vi "SwitchingCameraSendImagesToPCLoop.vi"(8 "error in (no error)":errorcluster, 9 "port":u16=1181, 10 "AutoSwitchCameraName":string="Sequenced Camera") -> ()   [LabVIEW 2019, in "ArgosLib.lvlib"]
doc: "This VI is used to serve images from one or more named cameras on your robot to the dashboard, SmartDashboard, or compatible web browser. Camera name and type info is published using network tables. Connections are on port 1181 by default and the URL for streaming can be found by looking at the network \"camera\"/streams variable. Cameras that are opened and stored in the name registry are automatically published by that name.\n\nThis VI runs in parallel with other code and should be placed in Robot Main or in Periodic Tasks.\n\nThis software is licensed. Open the labview\\readme\\WPI Robotics Library Open Source License.txt file for more information."
uses:
  ArgosLib.lvlib
  <vilib>/Rock Robotics/WPI/Utilities/Refnum Registry Operation.ctl
  <vilib>/Rock Robotics/Network Tables/NT Write String Array.vi
  <vilib>/Rock Robotics/Network Tables/NT Write String.vi
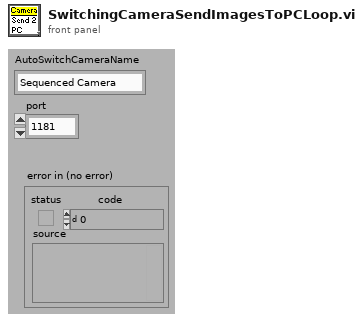
[diagram p1: front panel]
types:
  T1 = enum16{"Standard", "Buffered", "CRLF", "Immediate"}
  T2 = typedef "Refnum Registry Operation.ctl" = enum16{"set", "get", "delete", "get all names", "read name"}
  T3 = cluster{"token string":string, "token string 2":string}[]
  T4 = typedef "WPI_CameraDevRef.ctl" = cluster{"Camera Address":string, "CameraStatus":errorcluster}
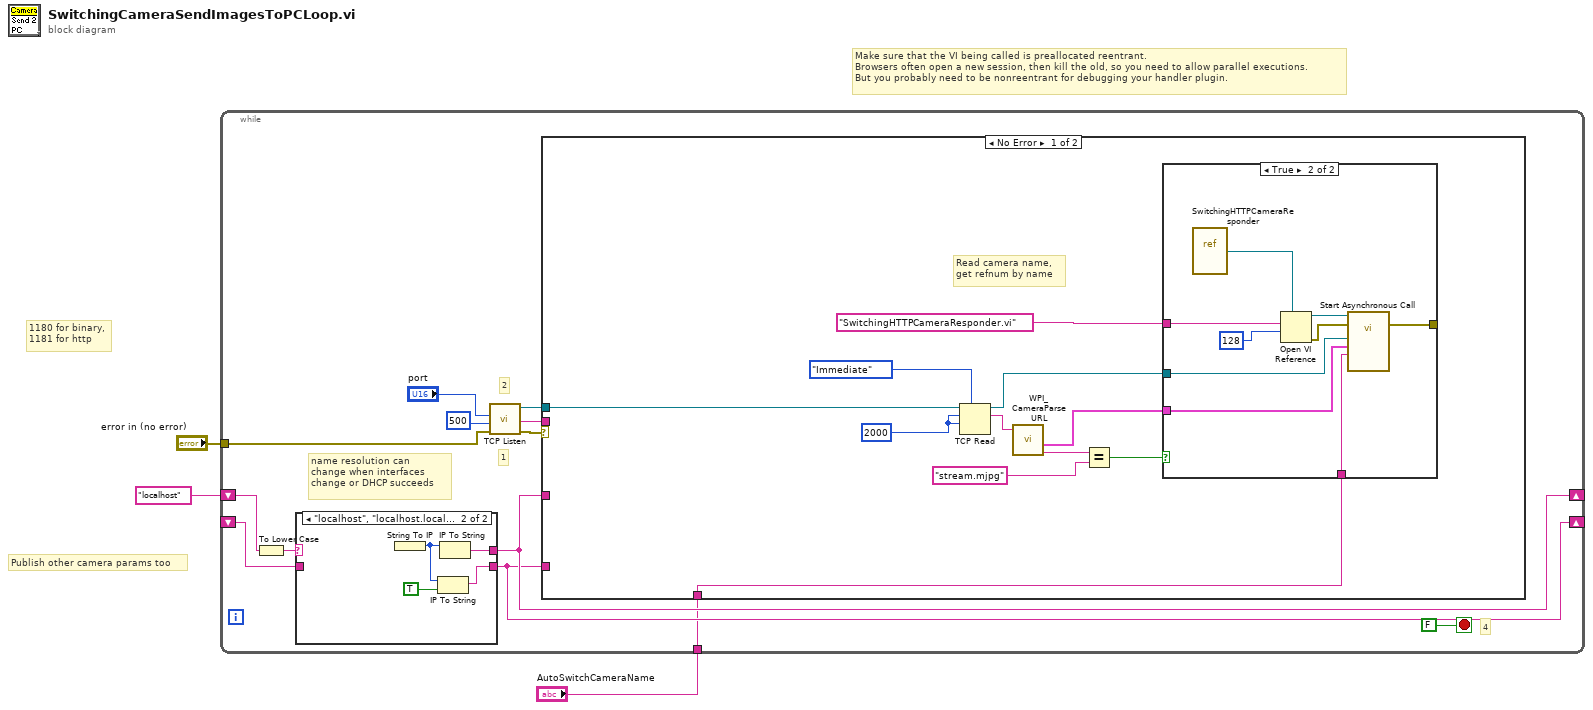
[diagram p0: block diagram]
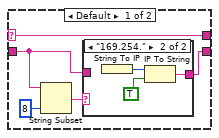
[diagram p2: hidden frame]
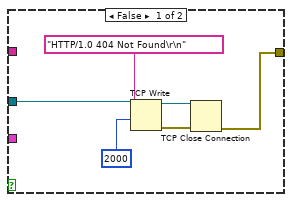
[diagram p4: hidden frame]
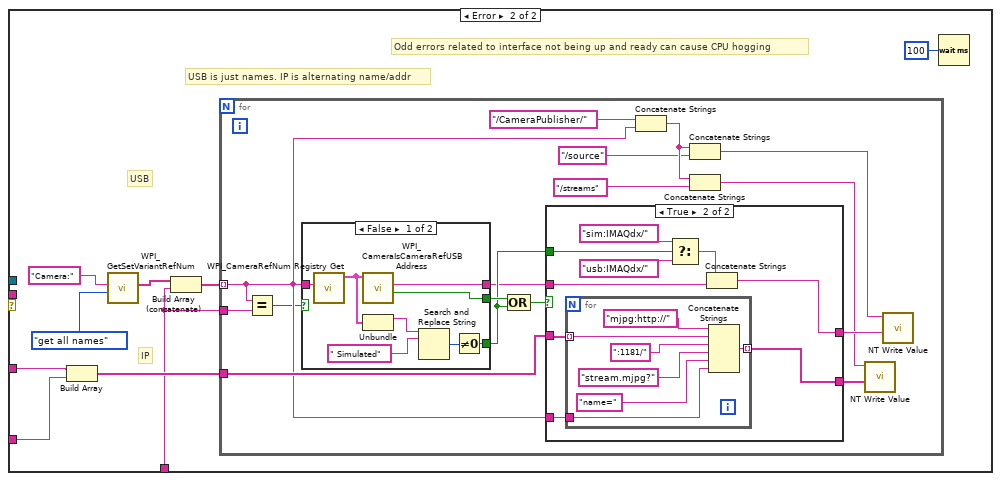
[diagram p5: hidden frame]
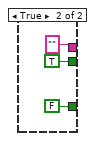
[diagram p6: hidden frame]
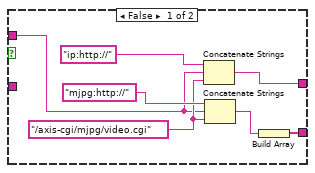
[diagram p7: hidden frame]
diagram:
  # "Make sure that the VI being called is preallocated reentrant.\nBrowsers often open a new session, then kill the old, so you need to allow parallel executions.\nBut you probably need to be nonreentrant for debugging your handler plugin."
  # "Publish other camera params too"
  # "1180 for binary,\n1181 for http"
  n1 = while {
    tunnel: "error in (no error)" -> [w15]
    shift-right: [w7] -> _
    shift-left: "localhost" -> [w8]
    shift-right: [w5] -> _
    shift-left: _ -> [w6]
    tunnel: "AutoSwitchCameraName" -> [w4]
    stop <- FALSE ("status") stop-if-true
    # "name resolution can\nchange when interfaces\nchange or DHCP succeeds"
    # "4"
    # "1"
    # "2"
    n2 = To Lower Case(string=w8) -> (all lower case string=w9:string)
    n3 = case shown="\"localhost\", \"localhost.localdomain\"" w9 {
      selector: w9 -> [w21 _]
      tunnel: [w21 w29] -> w7
      tunnel: w6 -> [w18 _]
      tunnel: [w17 w26] -> w5
      frame Default {
        n4 = String Subset(string=w18, length (rest)=8 ("length (rest)")) -> (substring=w19:string)  [unwired: 1 in]
        n5 = case shown="\"169.254.\"" w19 {
          tunnel: w18 -> [w22 _]
          tunnel: [w22 w23] -> w17
          frame Default {
          }
          frame "169.254." {
            n6 = String To IP() -> (0:w25:u32)  [unwired: 1 in]
            n7 = IP To String(1:TRUE ("dot notation? (F)"), 2:w25) -> (0:w23:string)
          }
        }
      }
      frame "localhost", "localhost.localdomain" {
        n8 = String To IP() -> (0:w27:u32)  [unwired: 1 in]
        n9 = IP To String(1:TRUE ("dot notation? (F)"), 2:w27) -> (0:w26:string)
        n10 = IP To String(2:w27) -> (0:w29:string)  [unwired: 1 in]
      }
    }
    n11 = call <vilib>:"TCP Listen.vi"("error in (no error)"=w15, "timeout ms (wait forever: -1)"=u16 500 ("port"), "port"="port") -> ("error out"=w12:errorcluster, "remote address"=w16:string, "connection ID"=w14:refnum<k5>)  [unwired: 1 in, 5 out]
    n12 = case shown="No Error" w12 {
      tunnel: w16 -> [_ _]
      tunnel: w14 -> [w37 _]
      tunnel: w7 -> [_ w61]
      tunnel: w5 -> [_ w59]
      tunnel: w4 -> [w30 w56]
      frame No Error {
        w38 = 2000
        # "Read camera name,\nget refnum by name"
        n13 = TCP Read(connection ID=w37, bytes to read=w38, 7:T1."Immediate" ("mode (standard)"), 9:w38) -> (connection ID out=w36:refnum<k5>, data out=w31:string)  [unwired: 1 in, 1 out]
        n14 = call <vilib>:"WPI_CameraParse URL.vi"("URL"=w31) -> ("cgi string"=w33:string, "parameters"=w32:T3)  [unwired: 7 in, 2 out]
        n15 = Equal?(x=w33, y="stream.mjpg") -> (x = y?=w35:bool)
        n16 = case shown="True" w35 {
          tunnel: "SwitchingHTTPCameraResponder.vi" -> [_ w55]
          tunnel: w36 -> [w46 w51]
          tunnel: [w41 w49] -> _
          tunnel: w32 -> [_ w48]
          tunnel: w30 -> [_ w47]
          frame False {
            n17 = TCP Write(connection ID=w46, data in="HTTP/1.0 404 Not Found\r\n" ("regular expression"), 9:2000) -> (connection ID out=w45:refnum<k5>, error out=w42:errorcluster)  [unwired: 1 in, 1 out]
            n18 = TCP Close Connection(connection ID=w45, error in (no error)=w42) -> (error out=w41:errorcluster)  [unwired: 2 out]
          }
          frame True {
            n19 = vi-ref "SwitchingHTTPCameraResponder.vi"() -> (w53:refnum<vi>)
            n20 = Open VI Reference(type specifier VI Refnum (for type only)=w53, vi path=w55, options=128) -> (vi reference=w52:refnum<vi>, error out=w50:errorcluster)  [unwired: 3 in]
            n21 = call-by-ref "Start Asynchronous Call"(reference=w52, error in=w50, "Switched Camera Name"=w47, "parameters"=w48, "connection ID"=w51) -> (error out=w49:errorcluster)  [unwired: 9 in, 1 out]
          }
        }
      }
      frame Error {
        # "USB is just names. IP is alternating name/addr"
        # "IP"
        # "USB"
        # "Odd errors related to interface not being up and ready can cause CPU hogging"
        n22 = Build Array(w61, w59) -> (w60:string[])
        n23 = call <vilib>:"WPI_GetSetVariantRefNum.vi"("Operation"=Refnum_Registry_Operation."get all names" ("menu"), "refnum name"="Camera:") -> ("names"=w58:string[])  [unwired: 7 in, 2 out]
        n24 = Build Array (concatenate)(w58, w56) -> (w57:string[])
        n25 = for {
          tunnel: w57 -> [w67] mode=indexing
          tunnel: w60 -> [w69]
          tunnel: w56 -> [w66]
          n26 = Equal?(x=w67, y=w66) -> (x = y?=w65:bool)
          n27 = case shown="False" w65 {
            tunnel: [w84 TRUE ("USB?")] -> w72
            tunnel: [w83 FALSE] -> w70
            tunnel: [w82 "" ("Camera Address Out")] -> w68
            tunnel: w67 -> [w81 _]
            frame False {
              n28 = call <vilib>:"WPI_CameraRefNum Registry Get.vi"("refnum name"=w81) -> ("CameraDevRef"=w87:T4)  [unwired: 9 in, 1 out]
              n29 = call <vilib>:"WPI_CameraIsCameraRefUSBAddress.vi"("CameraDevRef"=w87) -> ("USB?"=w84:bool, "Camera Address Out"=w82:string)  [unwired: 7 in, 2 out]
              n30 = Unbundle(w87) -> ("Camera Address"=w86:string)  [unwired: 1 out]
              n31 = Search and Replace String(input string=w86, search string=" Simulated") -> (number of replacements=w85:i32)  [unwired: 6 in, 3 out]
              n32 = Not Equal To 0?(x=w85) -> (x != 0?=w83:bool)
            }
            frame True {
            }
          }
          n33 = Compound Arithmetic op=OR(w72, w70) -> (w71:bool)
          n34 = case shown="True" w71 {
            tunnel: w68 -> [w94 w105]
            tunnel: w69 -> [_ w107]
            tunnel: w67 -> [_ w106]
            tunnel: [w92 w104] -> w80
            tunnel: [w96 w99] -> w73
            tunnel: w70 -> [_ w103]
            frame False {
              w95 = "/axis-cgi/mjpg/video.cgi"
              n35 = Concatenate Strings("ip:http://", w94, w95) -> (w92:string)
              n36 = Concatenate Strings("mjpg:http://", w94, w95) -> (w97:string)
              n37 = Build Array(w97) -> (w96:string[])
            }
            frame True {
              n38 = for {
                tunnel: w107 -> [w113] mode=indexing
                tunnel: w106 -> [w109]
                tunnel: [w108] -> w99 mode=indexing
                n39 = Concatenate Strings("mjpg:http://", w113, ":1181/", "stream.mjpg?", "name=", w109) -> (w108:string)
              }
              n40 = Select(t="sim:IMAQdx/", s=w103, f="usb:IMAQdx/") -> (s? t:f=w100:string)
              n41 = Concatenate Strings(w100, w105) -> (w104:string)
            }
          }
          n42 = Concatenate Strings("/CameraPublisher/", w67) -> (w77:string)
          n43 = Concatenate Strings(w77, "/source") -> (w74:string)
          n44 = Concatenate Strings(w77, "/streams") -> (w75:string)
          n45 = call-poly <vilib>:"NT Write Value.vi"("String Array"=w73, "Name"=w75) -> ()  [unwired: 9 in, 1 out]
          n46 = call-poly <vilib>:"NT Write Value.vi"("String"=w80, "Name"=w74) -> ()  [unwired: 9 in, 1 out]
        }
        n47 = Wait (ms)(milliseconds to wait=u32 100) -> ()  [unwired: 1 out]
      }
    }
  }
